vi "单个流程校验.vi"(5 "简易流程Id":u16(ring), 6 "是否是简易流程":bool, 7 "添加的路径":path, 8 "error in (no error)":errorcluster caption="错误输入（无错误）", 9 "量程":enum16{"低量程", "高量程"}(ring), 10 "测量模式":T1(ring), 11 "测量参数":u16(ring) items=["总氮"=2, "总磷"=1, "氨氮"=3, "COD"=22]) -> (0 "error out":errorcluster caption="错误输出", 2 "结果字符串":string, 3 "check？":bool)   [LabVIEW 2016, in "斯坦道氟化物.lvlib"]
uses:
  <vilib>/Plasmionique/MB Master/MB Master.lvlib
panel:
  out "数组":u16[](array[numeric])
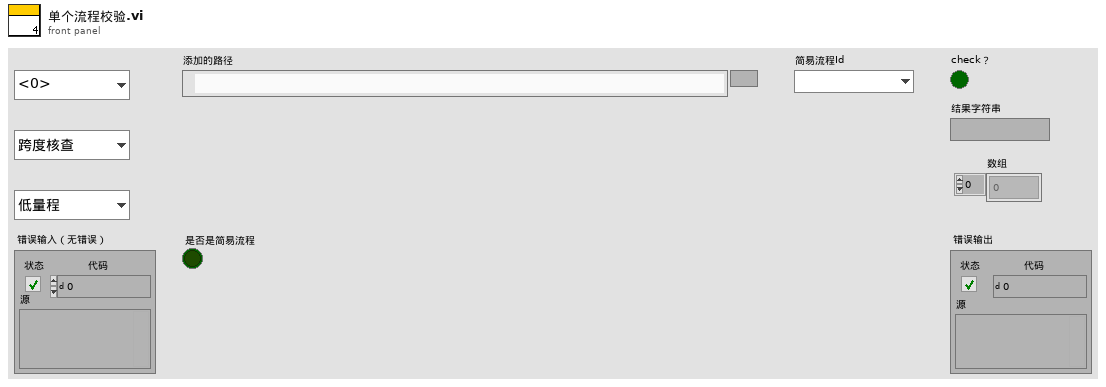
[diagram p1: front panel]
types:
  T1 = enum16{"跨度核查", "水样测量", "零点核查", "标样核查", "加标回收", "快捷测试", "空白校准", "标样校准"}
  T2 = cluster{"测量参数":u16, "测量模式":enum16{"跨度核查", "水样测量", "零点核查", "标样核查", "加标回收", "快捷测试", "空白校准", "标样校准"}, "量程":enum16{"低量程", "高量程"}}
  T3 = cluster{"port":i32, "dac":u8, "adc":u8, "time":u16, "步骤名":string}[]
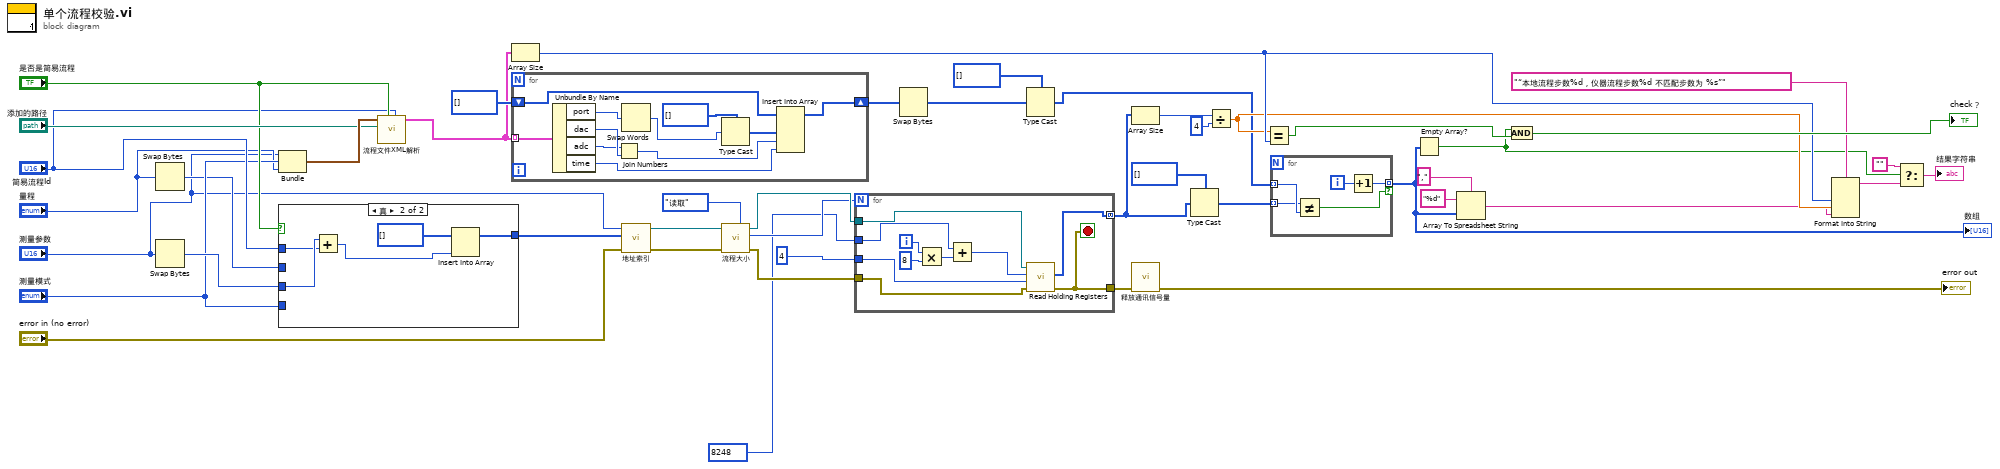
[diagram p0: block diagram]
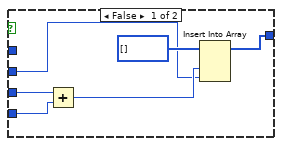
[diagram p2: hidden frame]
diagram:
  n1 = Swap Bytes(anything="量程") -> (byte swapped=w36:u16)
  n2 = Swap Bytes(anything="测量参数") -> (byte swapped=w40:u16)
  n3 = Bundle("测量参数"="测量参数", "测量模式"="测量模式", "量程"="量程") -> (w45:T2)  [unwired: 1 in]
  n4 = case shown="真" "是否是简易流程" {
    tunnel: [w49 w54] -> w34
    tunnel: "测量模式" -> [w48 _]
    tunnel: w40 -> [w47 w53]
    tunnel: w36 -> [w46 _]
    tunnel: "简易流程Id" -> [_ w52]
    frame False {
      n5 = Add(x=w47, y=w48) -> (x+y=w51:u16)
      n6 = Insert Into Array(array=u16[] [] ("数组"), new element #1=w51, new element #2=w46) -> (w49:u16[])  [unwired: 1 in]
    }
    frame True {
      n7 = Add(x=w53, y=w52) -> (x+y=w56:u16)
      n8 = Insert Into Array(array=u16[] [] ("数组"), new element=w56) -> (w54:u16[])  [unwired: 1 in]
    }
  }
  n9 = call "流程文件XML解析.vi"("简易流程Id"="简易流程Id", "是否是简易流程"="是否是简易流程", "添加的路径"="添加的路径", "参数簇"=w45) -> ("数组"=w41:T3)  [unwired: 7 in]
  n10 = Array Size(array=w41) -> (size(s)=w17:i32)
  n11 = for {
    tunnel: w41 -> [w67] mode=indexing
    shift-right: [w62] -> w42
    shift-left: u16[] [] -> [w60]
    n12 = Unbundle By Name(w67) -> ("port"=w65:i32, "dac"=w58:u8, "adc"=w57:u8, "time"=w63:u16)
    n13 = Join Numbers(hi=w57, lo=w58) -> ((hi.lo)=w64:u16)
    n14 = Swap Words(1:w65) -> (0:w59:i32)
    n15 = Type Cast(type=u16[] [], x=w59) -> (*(type *) &x=w61:u16[])
    n16 = Insert Into Array(array=w60, new element #1=w61, new element #2=w64, new element #3=w63) -> (w62:u16[])  [unwired: 1 in]
  }
  n17 = call "地址索引.vi"("error in (no error)"="error in (no error)", "values"=w34, "测量参数"="测量参数") -> ("error out"=w31:errorcluster, "MB session out"=w30:refnum<class "MB_Master.lvclass">)  [unwired: 7 in]
  n18 = call "流程大小.vi"("功能"=enum16{"写入", "读取"}."读取", "error in (no error)"=w31, "MB session in"=w30) -> ("error out"=w28:errorcluster, "大小读取"=w16:i32, "MB session out"=w29:refnum<class "MB_Master.lvclass">)  [unwired: 6 in]
  n19 = for {
    N: w16 -> [_]
    tunnel: u16 8248 ("starting address") -> [w77]
    tunnel: [w70] -> w27
    tunnel: w29 -> [w73]
    tunnel: w28 -> [w72]
    tunnel: [w69] -> w4 mode=concatenating
    tunnel: 4 ("y") -> [w68]
    i -> [w74]
    stop <- w70 stop-if-true
    n20 = Multiply(x=w74, y=8) -> (x*y=w76:i32)
    n21 = Add(x=w77, y=w76) -> (x+y=w71:i32)
    n22 = call <vilib>:"Read Holding Registers.vi"("error in (no error)"=w72, "quantity"=w68, "starting address"=w71, "MB session in"=w73) -> ("error out"=w70:errorcluster, "Registers"=w69:u16[])  [unwired: 5 in, 1 out]
  }
  n23 = Swap Bytes(anything=w42) -> (byte swapped=w24:u16[])
  n24 = Type Cast(type=u64[] [], x=w24) -> (*(type *) &x=w7:u64[])
  n25 = Array Size(array=w4) -> (size(s)=w14:i32)
  n26 = call "释放通讯信号量.vi"("error in (no error)"=w27) -> ("error out"=→"error out":errorcluster)  [unwired: 10 in]
  n27 = Type Cast(type=u64[] [], x=w4) -> (*(type *) &x=w5:u64[])
  n28 = Divide(x=w14, y=4) -> (x/y=w15:dbl)
  n29 = Equal?(x=w15, y=w17) -> (x = y?=w23:bool)
  n30 = for {
    tunnel: w5 -> [w81] mode=indexing
    tunnel: w7 -> [w82] mode=indexing
    tunnel: [w78] -> w2 mode=indexing if=w80
    i -> [w79]
    n31 = Not Equal?(x=w81, y=w82) -> (x != y?=w80:bool)
    n32 = Increment(x=w79) -> (x+1=w78:i32)
  }
  "数组" <- w2
  n33 = Empty Array?(array=w2) -> (empty?=w11:bool)
  n34 = Array To Spreadsheet String(delimiter (Tab)="," ("分隔符(Tab)"), array=w2, 3:"%d" ("格式字符串")) -> (spreadsheet string=w12:string)
  n35 = And(x=w11, y=w23) -> (x .and. y?=→"check？":bool)
  n36 = Format Into String(format string="“本地流程步数%d，仪器流程步数%d 不匹配步数为 %s”" ("格式字符串"), w17, w15, w12) -> (resulting string=w10:string)  [unwired: 2 in, 1 out]
  n37 = Select(t="", s=w11, f=w10) -> (s? t:f=→"结果字符串":string)
